vi "Verify Parameterized.vi"(5 "Options":T1, 7 "Test VI (caller)":string, 8 "error in":errorcluster, 9 "Set (map: control name  -> value as variant)":set{map{string, variant}}(c389), 10 "VI Refnum":refnum<vi>) -> (0 "error out":errorcluster)   [LabVIEW 2020, in "Caraya.Extension.lvlib"]
uses:
  Approval Tests/Options.ctl
  Approval Tests/Reporter/Reporter.lvclass
  Approval Tests/Printer/Printer.lvclass
  <vilib>/addons/_JKI Toolkits/Caraya/classes/Assert/Assert True.vi
  Caraya.Extension.lvlib
  <vilib>/addons/_JKI Toolkits/Caraya/classes/Assert/Assert.lvclass
  Approval Tests/Approval Tests.lvlib
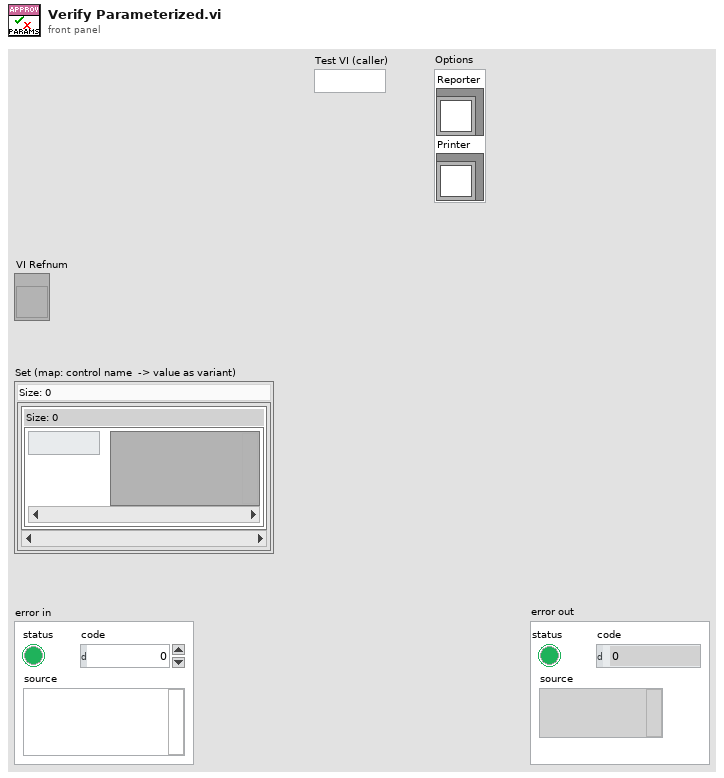
[diagram p1: front panel]
types:
  T1 = typedef "Approval Tests.lvlib/Options.ctl" = cluster{"Reporter":refnum<class "Reporter.lvclass">, "Printer":refnum<class "Printer.lvclass">}
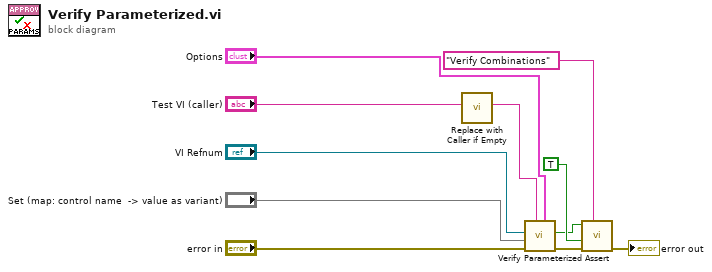
[diagram p0: block diagram]
diagram:
  n1 = call "Replace with Caller if Empty.vi"("Test VI (caller) in"="Test VI (caller)") -> ("Test VI (caller) out"=w4:string)  [unwired: 10 in]
  n2 = call "Verify Parameterized.vi"("Options"="Options", "Test VI (caller)"=w4, "error in"="error in", "Set (map: control name  -> value as variant)"="Set (map: control name  -> value as variant)", "VI in"="VI Refnum") -> ("error out"=w9:errorcluster, "Passed?"=w2:bool)  [unwired: 4 in, 1 out]
  n3 = call-poly <vilib>:"Assert.vi"("Label"="Verify Combinations", "error in (no error)"=w9, "Register with caller test (F)"=TRUE, "True?"=w2) -> ("error out"=→"error out":errorcluster)  [unwired: 6 in, 1 out]
